vi "Update Elevator State.vi"(8 "error in (no error)":errorcluster, 10 "Elevator State":T1 {"Current Elevation" scale=0.0..100.0; "Current Travel Rate" scale=-1.0..1.0}, 11 "Elevator State Receiver in":refnum<class "Elevator State Receiver.lvclass">) -> (0 "error out":errorcluster, 3 "Elevator State Receiver out":refnum<class "Elevator State Receiver.lvclass">)   [LabVIEW 2014, in "Elevator.lvlib" / "Elevator State Receiver.lvclass"]
uses:
  Elevator State Receiver.lvclass
  Elevator Class/Elevator State.ctl
  Elevator State Receiver.lvclass/Elevator State Receiver.ctl
  Elevator Class/Elevator.lvclass
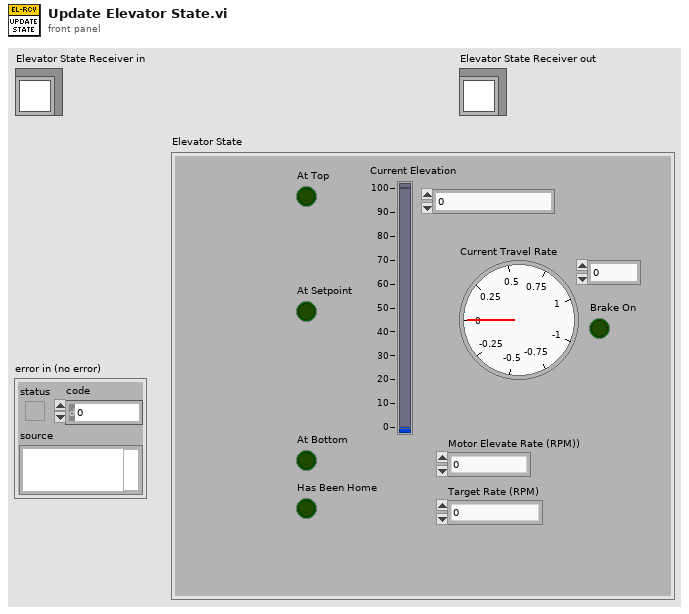
[diagram p1: front panel]
types:
  T1 = typedef "Elevator.lvlib/Elevator.lvclass/Elevator State.ctl" = cluster{"At Bottom":bool, "At Top":bool, "At Setpoint":bool, "Target Rate (RPM)":dbl, "Current Travel Rate":dbl, "Current Elevation":dbl, "Brake On":bool, "Motor Elevate Rate (RPM))":dbl, "Has Been Home":bool}
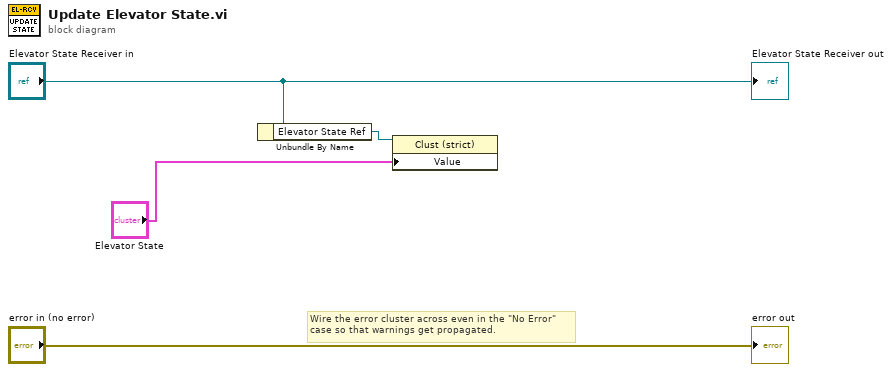
[diagram p0: block diagram]
diagram:
  # "Wire the error cluster across even in the \"No Error\"\ncase so that warnings get propagated."
  n1 = Unbundle By Name("Elevator State Receiver in") -> ("Elevator State Ref"=w2:refnum<vi>)
  n2 = property class="Clust (strict)"(reference=w2, "Value"="Elevator State") -> ()  [unwired: 1 in, 2 out]
  "error out" <- "error in (no error)"
  "Elevator State Receiver out" <- "Elevator State Receiver in"
